vi "Initialization VI.vi"(8 "error in":errorcluster, 10 "Custom XML":string, 11 "Item Ref in":u64 format="%.0x") -> (0 "error out":errorcluster, 3 "Item Ref out":u64 format="%.0x")   [LabVIEW 2026, in "Template Configuration.lvlib"]
uses:
  Template Configuration.lvlib
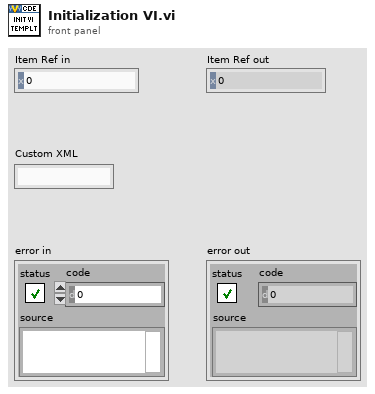
[diagram p1: front panel]
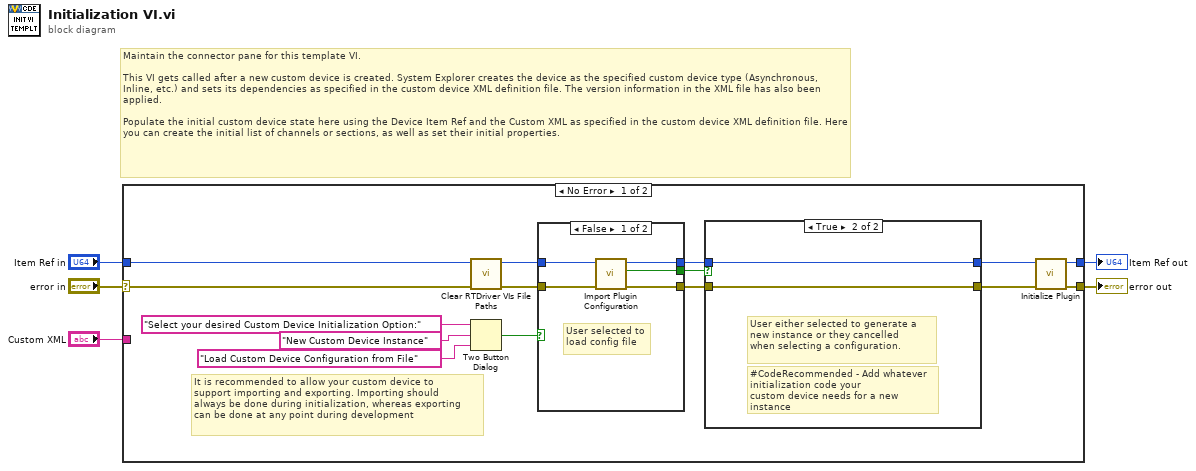
[diagram p0: block diagram]
diagram:
  # "Maintain the connector pane for this template VI.\n\nThis VI gets called after a new custom device is created. System Explorer creates the device as the specified custom device type (Asynchronous, Inline, etc.) and sets its dependencies as specified in the custom device XML definition file. The version information in the XML file has also been applied.\n\nPopulate the initial custom device state here using the Device Item Ref and the Custom XML as specified in the custom device XML definition file. Here you can create the initial list of channels or sections, as well as set their initial properties."
  n1 = case shown="No Error" "error in" {
    selector: "error in" -> [w20 w34]
    tunnel: [w19 w34] -> w5
    tunnel: [w17 w33] -> w3
    tunnel: "Item Ref in" -> [w18 w33]
    tunnel: "Custom XML" -> [_ _]
    frame No Error {
      # "It is recommended to allow your custom device to\nsupport importing and exporting. Importing should\nalways be done during initialization, whereas exporting\ncan be done at any point during development"
      n2 = call "Clear RTDriver VIs File Paths.vi"("error in"=w20, "Item Ref in"=w18) -> ("error out"=w15:errorcluster, "Item Ref out"=w8:u64)  [unwired: 8 in]
      n3 = Two Button Dialog(message="Select your desired Custom Device Initialization Option:", 1:"Load Custom Device Configuration from File" ("F button name (\"Cancel\")"), 2:"New Custom Device Instance" ("T button name (\"OK\")")) -> (T button?=w11:bool)
      n4 = case "New or Load" shown="False" w11 {
        selector: w11 -> [_ w30]
        tunnel: w8 -> [w29 w31]
        tunnel: [w27 w31] -> w10
        tunnel: w15 -> [w28 w32]
        tunnel: [w25 w32] -> w16
        tunnel: [w26 w30] -> w9
        frame False {
          # "User selected to\nload config file"
          n5 = call "Import Plugin Configuration.vi"("error in"=w28, "Item Ref in"=w29) -> ("error out"=w25:errorcluster, "cancelled"=w26:bool, "Item Ref out"=w27:u64)  [unwired: 7 in]
        }
        frame True {
          # "User selected new\ncustom device. Do\nnothing in this case\nand handle new\ngeneration in the\nnext case structure"
        }
      }
      n6 = case "Create New" shown="True" w9 {
        tunnel: w10 -> [w21 w23]
        tunnel: w16 -> [w22 w24]
        tunnel: [w22 w24] -> w6
        tunnel: [w21 w23] -> w7
        frame False {
          # "User selected to import from configuration and didn't cancel import"
        }
        frame True {
          # "#CodeRecommended - Add whatever initialization code your\ncustom device needs for a new instance"
          # "User either selected to generate a new instance or they cancelled\nwhen selecting a configuration."
        }
      }
      n7 = call "Initialize Plugin.vi"("error in"=w6, "Item Ref in"=w7) -> ("error out"=w19:errorcluster, "Item Ref out"=w17:u64)  [unwired: 8 in]
    }
    frame Error {
    }
  }
  "error out" <- w5
  "Item Ref out" <- w3
